vi "Log Event.vi"(9 "Message":string, 10 "Log Level":T1) -> (2 "All Events":string[](array[string]))   [LabVIEW 2019]
uses:
  Log Level.ctl
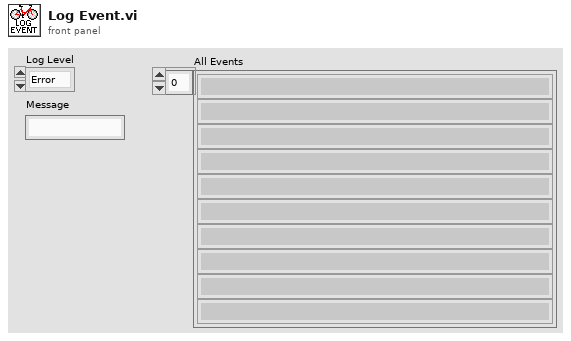
[diagram p1: front panel]
types:
  T1 = typedef "Log Level.ctl" = enum16{"Error", "Warning", "Info"}
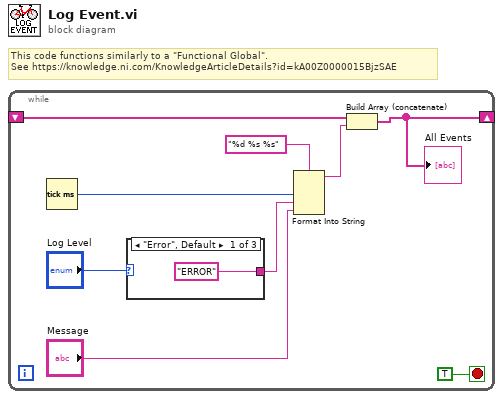
[diagram p0: block diagram]
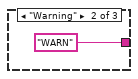
[diagram p2: hidden frame]
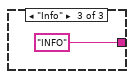
[diagram p3: hidden frame]
diagram:
  # "This code functions similarly to a \"Functional Global\".\nSee https://knowledge.ni.com/KnowledgeArticleDetails?id=kA00Z0000015BjzSAE"
  n1 = while {
    shift-right: [w8] -> _
    shift-left: _ -> [w7]
    stop <- TRUE stop-if-true
    n2 = Tick Count (ms)() -> (millisecond timer value=w5:u32)
    n3 = case shown="\"Error\", Default" "Log Level" {
      tunnel: ["ERROR" "WARN" "INFO"] -> w2
      frame "Error", Default {
      }
      frame "Warning" {
      }
      frame "Info" {
      }
    }
    n4 = Format Into String(format string="%d %s %s", w5, w2, "Message") -> (resulting string=w1:string)  [unwired: 2 in, 1 out]
    n5 = Build Array (concatenate)(w7, w1) -> (w8:string[])
    "All Events" <- w8
  }
